vi "ElevatorStateSelect.vi"() -> (2 "Elevator State":string)   [LabVIEW 2018]
uses:
  Inputs_DriverStation.vi
  RobotStates.vi
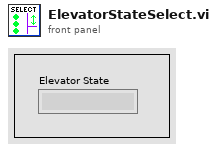
[diagram p1: front panel]
types:
  T1 = cluster{"Elevator_Stow":bool, "Cargo_Ground":bool, "Cargo_Feeder":bool, "Cargo_Ship":bool, "Cargo_Rocket_1":bool, "Cargo_Rocket_2":bool, "Cargo_Rocket_3":bool, "Hatch_Ground":bool, "Hatch_Feeder":bool, "Hatch_Ship":bool, "Hatch_Rocket_1":bool, "Hatch_Rocket_2":bool, "Hatch_Rocket_3":bool, "Climb":bool}
  T2 = cluster{"Trigger":bool, "Trigger":bool, "Trigger":bool, "Trigger":bool, "Trigger":bool, "Trigger":bool, "Trigger":bool, "Trigger":bool, "Trigger":bool, "Trigger":bool, "Trigger":bool, "Trigger":bool, "Trigger":bool, "Trigger":bool}
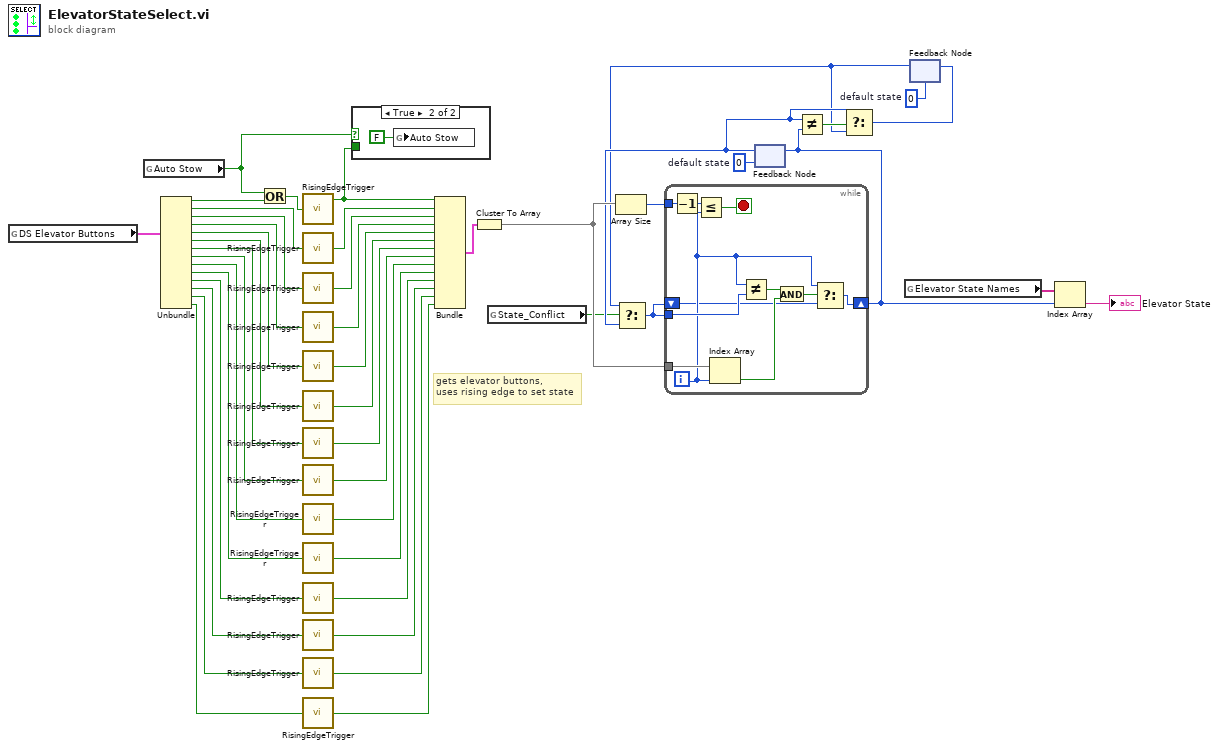
[diagram p0: block diagram]
diagram:
  w5 = 0  # default state
  w44 = 0  # default state
  # "gets elevator buttons,\nuses rising edge to set state"
  n1 = global read "Inputs_DriverStation.vi" "DS Elevator Buttons"() -> (w39:T1)
  n2 = global read "RobotStates.vi" "Auto Stow"() -> (w10:bool)
  n3 = Unbundle(w39) -> ("Elevator_Stow"=w11:bool, "Cargo_Ground"=w41:bool, "Cargo_Feeder"=w40:bool, "Cargo_Ship"=w36:bool, "Cargo_Rocket_1"=w35:bool, "Cargo_Rocket_2"=w34:bool, "Cargo_Rocket_3"=w33:bool, "Hatch_Ground"=w28:bool, "Hatch_Feeder"=w27:bool, "Hatch_Ship"=w26:bool, "Hatch_Rocket_1"=w25:bool, "Hatch_Rocket_2"=w24:bool, "Hatch_Rocket_3"=w23:bool, "Climb"=w14:bool)
  n4 = Or(x=w10, y=w11) -> (x .or. y?=w12:bool)
  n5 = call "RisingEdgeTrigger.vi"("Raw Signal"=w12) -> ("Trigger"=w9:bool)
  n6 = call "RisingEdgeTrigger.vi"("Raw Signal"=w41) -> ("Trigger"=w43:bool)
  n7 = call "RisingEdgeTrigger.vi"("Raw Signal"=w40) -> ("Trigger"=w42:bool)
  n8 = call "RisingEdgeTrigger.vi"("Raw Signal"=w36) -> ("Trigger"=w32:bool)
  n9 = call "RisingEdgeTrigger.vi"("Raw Signal"=w35) -> ("Trigger"=w31:bool)
  n10 = call "RisingEdgeTrigger.vi"("Raw Signal"=w34) -> ("Trigger"=w30:bool)
  n11 = call "RisingEdgeTrigger.vi"("Raw Signal"=w33) -> ("Trigger"=w29:bool)
  n12 = call "RisingEdgeTrigger.vi"("Raw Signal"=w28) -> ("Trigger"=w22:bool)
  n13 = call "RisingEdgeTrigger.vi"("Raw Signal"=w27) -> ("Trigger"=w21:bool)
  n14 = call "RisingEdgeTrigger.vi"("Raw Signal"=w26) -> ("Trigger"=w20:bool)
  n15 = call "RisingEdgeTrigger.vi"("Raw Signal"=w25) -> ("Trigger"=w19:bool)
  n16 = call "RisingEdgeTrigger.vi"("Raw Signal"=w24) -> ("Trigger"=w18:bool)
  n17 = call "RisingEdgeTrigger.vi"("Raw Signal"=w23) -> ("Trigger"=w17:bool)
  n18 = call "RisingEdgeTrigger.vi"("Raw Signal"=w14) -> ("Trigger"=w13:bool)
  n19 = case shown="True" w10 {
    tunnel: w9 -> [_ _]
    frame False {
    }
    frame True {
      n20 = global write "RobotStates.vi" "Auto Stow"(FALSE ("Auto Stow")) -> ()
    }
  }
  n21 = Bundle("Trigger"=w9, "Trigger"=w43, "Trigger"=w42, "Trigger"=w32, "Trigger"=w31, "Trigger"=w30, "Trigger"=w29, "Trigger"=w22, "Trigger"=w21, "Trigger"=w20, "Trigger"=w19, "Trigger"=w18, "Trigger"=w17, "Trigger"=w13) -> (w16:T2)  [unwired: 1 in]
  n22 = Cluster To Array(cluster=w16) -> (array=w45:bool[])
  n23 = global read "RobotStates.vi" "State_Conflict"() -> (w1:bool)
  n24 = Array Size(array=w45) -> (size(s)=w15:i32)
  n25 = feedback #1(w44) -> (w4:i32)
  n26 = global read "RobotStates.vi" "Elevator State Names"() -> (w38:string[])
  n27 = feedback #2(w5) -> (w2:i32)
  n28 = Select(t=w2, s=w1, f=w4) -> (s? t:f=w3:i32)
  n29 = while {
    tunnel: w45 -> [w57]
    tunnel: w3 -> [w52]
    tunnel: w15 -> [w50]
    shift-right: [w53] -> w8
    shift-left: w3 -> [w47]
    i -> [w51]
    stop <- w49 stop-if-true
    n30 = Decrement(x=w50) -> (x-1=w48:i32)
    n31 = Less Or Equal?(x=w48, y=w51) -> (x <= y?=w49:bool)
    n32 = Index Array(array=w57, index=w51) -> (element=w55:bool)
    n33 = Not Equal?(x=w51, y=w52) -> (x != y?=w54:bool)
    n34 = And(x=w54, y=w55) -> (x .and. y?=w56:bool)
    n35 = Select(t=w51, s=w56, f=w47) -> (s? t:f=w53:i32)
  }
  n36 = feedback-in #1(w8) -> ()
  n37 = Not Equal?(x=w4, y=w8) -> (x != y?=w7:bool)
  n38 = Select(t=w4, s=w7, f=w2) -> (s? t:f=w6:i32)
  n39 = feedback-in #2(w6) -> ()
  n40 = Index Array(array=w38, index=w8) -> (element=→"Elevator State":string)
